vi "Get Table Values Range.vi"(7 "Sheet Name in":string, 8 "error in":errorcluster, 10 "Table Name":string, 11 "SpreadsheetDoc in":refnum<k24>) -> (0 "error out":errorcluster, 2 "Range":string, 3 "SpreadsheetDoc out":refnum<k24>, 5 "Sheet Name out":string)   [LabVIEW 2019, in "Open Xml.lvlib"]
uses:
  Open Xml.lvlib
  D:/git/Open-Xml-LabVIEW/Source/DocumentFormat.OpenXml.dll
  DocumentFormat.OpenXml.dll
  D:/git/Open-Xml-LabVIEW/Source/DocumentFormat.OpenXml.Framework.dll
  DocumentFormat.OpenXml.Framework.dll
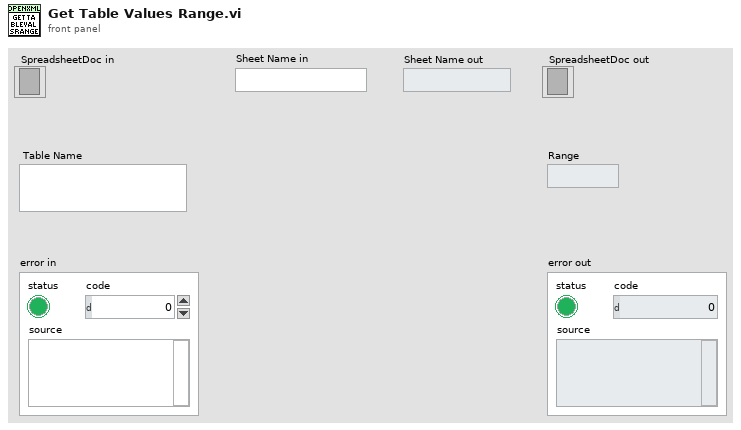
[diagram p1: front panel]
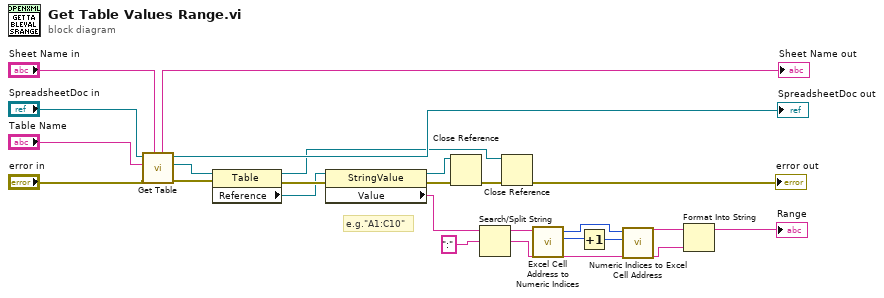
[diagram p0: block diagram]
diagram:
  # "e.g.\"A1:C10\""
  n1 = call "Get Table.vi"("Sheet Name in"="Sheet Name in", "error in"="error in", "Table Name"="Table Name", "SpreadsheetDoc in"="SpreadsheetDoc in") -> ("error out"=w18:errorcluster, "Table"=w9:refnum<k24>, "SpreadsheetDoc out"=→"SpreadsheetDoc out":refnum<k24>, "Sheet Name out"=→"Sheet Name out":string)  [unwired: 4 in]
  n2 = property class="Table"(reference=w9, error in=w18) -> (reference out=w10:refnum<k24>, error out=w21:errorcluster, "Reference"=w20:refnum<k24>)
  n3 = property class="StringValue"(reference=w20, error in=w21) -> (reference out=w19:refnum<k24>, error out=w24:errorcluster, "Value"=w22:string)
  n4 = Close Reference(reference=w19, error in (no error)=w24) -> (error out=w23:errorcluster)
  n5 = Search/Split String(string=w22, search string/char (-)=":") -> (substring before match=w7:string, match + rest of string=w2:string)  [unwired: 1 in, 1 out]
  n6 = Close Reference(reference=w10, error in (no error)=w23) -> (error out=→"error out":errorcluster)
  n7 = call "Excel Cell Address to Numeric Indices.vi"("Cell Name"=w7) -> ("Row Number"=w6:i32, "Column Number"=w4:i32)  [unwired: 9 in]
  n8 = Increment(x=w6) -> (x+1=w5:i32)
  n9 = call "Numeric Indices to Excel Cell Address.vi"("Row"=w5, "Column"=w4) -> ("Cell Address"=w3:string)  [unwired: 9 in]
  n10 = Format Into String(initial string=w3, w2) -> (resulting string=→"Range":string)  [unwired: 2 in, 1 out]
